vi "LATLONG to bearing.vi"(8 "LONG2":dbl, 9 "LAT2":dbl, 10 "LONG1":dbl, 11 "LAT1":dbl) -> (1 "Y":dbl, 2 "X":dbl, 3 "Bearing (deg)":dbl)   [LabVIEW 2015]
uses:
  <vilib>/imath/engines/lvmath2/RunTimeEngine/BuiltInFunctions/atan2/NIMS_atan2.vi
  <instcachedir>/0/NIMS_atan2_A91AA4A7D42247EDBE8F76DB99AF04A4.lvgen/NIMS_atan2_A91AA4A7D42247EDBE8F76DB99AF04A4_000.vi
  <vilib>/imath/engines/lvmath2/RunTimeEngine/NodeEndStatement/NIMS_NodeEndStatement_Output.vi
  <instcachedir>/0/NIMS_NodeEndStatement_Output_53EC0D466D134D7ABD903AC30B43404B.lvgen/NIMS_NodeEndStatement_Output_53EC0D466D134D7ABD903AC30B43404B_001.vi
  <vilib>/imath/engines/lvmath2/RunTimeEngine/ErrorHandling/NIMS_Finalize Error.vi
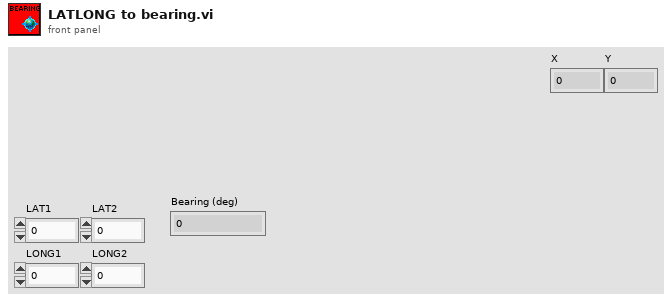
[diagram p1: front panel]
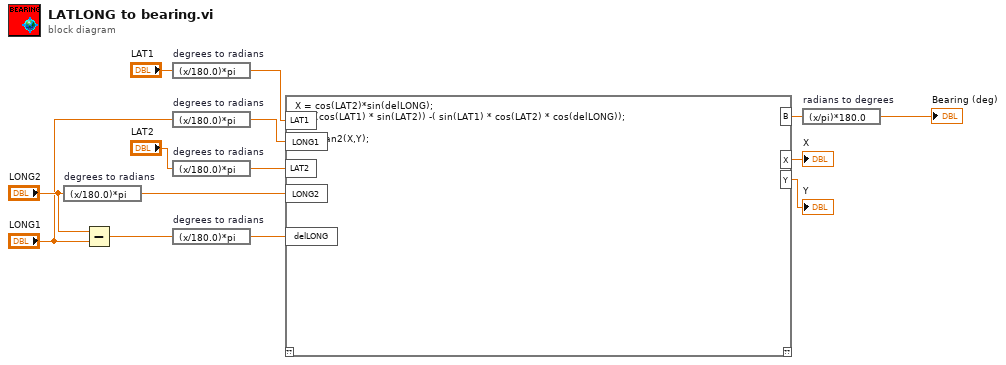
[diagram p0: block diagram]
diagram:
  n1 = expression code="(x/180.0)*pi" "degrees to radians"("LONG2") -> (w14:dbl)
  n2 = Subtract(x="LONG2", y="LONG1") -> (x-y=w10:dbl)
  n3 = expression code="(x/180.0)*pi" "degrees to radians"("LAT1") -> (w13:dbl)
  n4 = expression code="(x/180.0)*pi" "degrees to radians"("LONG1") -> (w12:dbl)
  n5 = expression code="(x/180.0)*pi" "degrees to radians"("LAT2") -> (w11:dbl)
  n6 = expression code="(x/180.0)*pi" "degrees to radians"(w10) -> (w9:dbl)
  n7 = mathscript code="X = cos(LAT2)*sin(delLONG);\nY = (cos(LAT1) * sin(LAT2)) -( sin(LAT1) * cos(LAT2) * cos(delLONG));\n\nB = atan2(X,Y);"("LAT1"=w13, "LONG1"=w12, "LAT2"=w11, "LONG2"=w14, "delLONG"=w9) -> ("B"=w8:dbl, "X"=→"X":dbl, "Y"=→"Y":dbl)  [unwired: 1 in, 1 out]
  n8 = expression code="(x/pi)*180.0" "radians to degrees"(w8) -> (→"Bearing (deg)":dbl)
